vi "Send HELLO.vi"(8 "error in (no error)":errorcluster, 11 "WAMP Client in":refnum<class "WAMP Client.lvclass">) -> (0 "error out":errorcluster, 3 "WAMP Client out":refnum<class "WAMP Client.lvclass">)   [LabVIEW 2020, in "wamplv.lvlib" / "WAMP Client.lvclass"]
uses:
  WAMP Client.lvclass
  WAMP Client.lvclass/WAMP Client.ctl
  Private/Comm Handlers/ICommHandler/ICommHandler.lvclass
  Private/Authenticators/IAuthenticator/IAuthenticator.lvclass
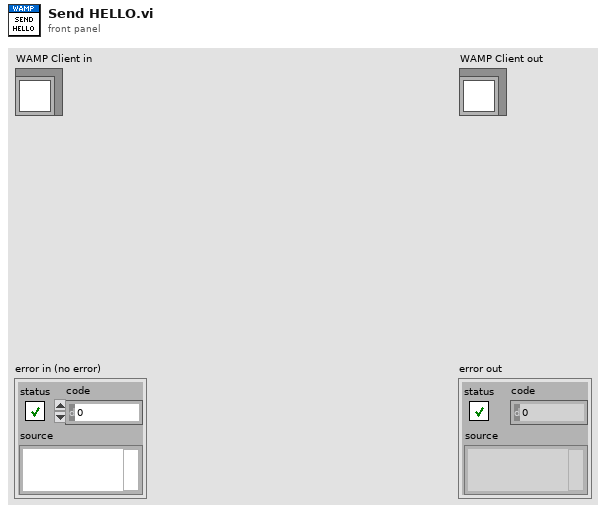
[diagram p1: front panel]
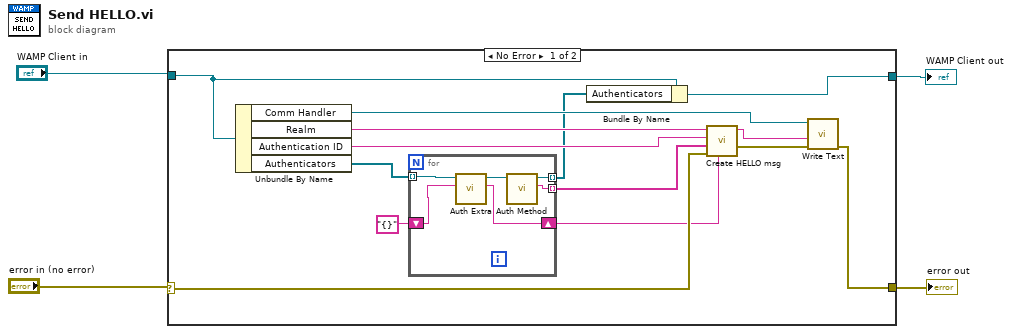
[diagram p0: block diagram]
diagram:
  n1 = case shown="No Error" "error in (no error)" {
    selector: "error in (no error)" -> [w15 w26]
    tunnel: [w13 w26] -> w3
    tunnel: [w7 w25] -> w1
    tunnel: "WAMP Client in" -> [w8 w25]
    frame No Error {
      n2 = Unbundle By Name(w8) -> ("Comm Handler"=w18:refnum<class "ICommHandler.lvclass">, "Realm"=w17:string, "Authentication ID"=w10:string, "Authenticators"=w12:refnum<class "IAuthenticator.lvclass">[])
      n3 = for {
        tunnel: w12 -> [w23] mode=indexing
        tunnel: [w24] -> w11 mode=indexing
        tunnel: [w21] -> w6 mode=indexing
        shift-right: [w20] -> w5
        shift-left: "{}" -> [w19]
        n4 = call-dynamic "Auth Extra.vi"("authextra in"=w19, "IAuthenticator in"=w23) -> ("authextra"=w20:string, "IAuthenticator out"=w22:refnum<class "IAuthenticator.lvclass">)  [unwired: 7 in, 1 out]
        n5 = call-dynamic "Auth Method.vi"("IAuthenticator in"=w22) -> ("Authmethod"=w24:string, "IAuthenticator out"=w21:refnum<class "IAuthenticator.lvclass">)  [unwired: 9 in]
      }
      n6 = Bundle By Name(cluster=w8, "Authenticators"=w6) -> (w7:refnum<class "WAMP Client.lvclass">)
      n7 = call "Create HELLO msg.vi"("aututhextras"=w5, "error in (no error)"=w15, "Authmethods"=w11, "Auth ID"=w10, "Realm"=w17) -> ("error out"=w14:errorcluster, "WAMP message"=w16:string)  [unwired: 5 in]
      n8 = call-dynamic "Write Text.vi"("error in (no error)"=w14, "String"=w16, "ICommHandler in"=w18) -> ("error out"=w13:errorcluster)  [unwired: 7 in, 1 out]
    }
    frame Error {
    }
  }
  "error out" <- w3
  "WAMP Client out" <- w1
